vi "getDeviceParam.vi"(9 "deviceNo":i32, 10 "param":string, 11 "driver":string) -> (3 "Result":string)   [LabVIEW 2015]
uses:
  <instrlib>/niModInst/niModInst Get Installed Device Attribute (String).vi
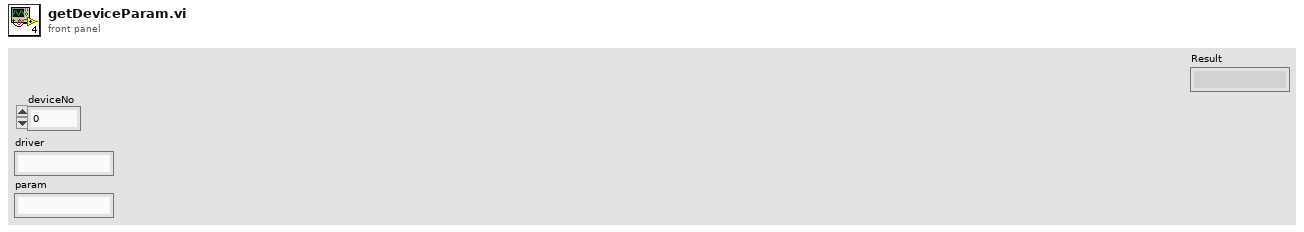
[diagram p1: front panel]
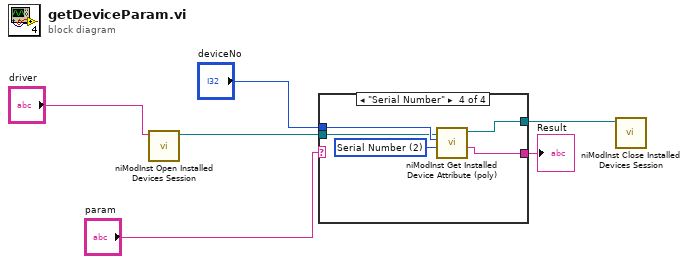
[diagram p0: block diagram]
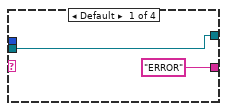
[diagram p2: hidden frame]
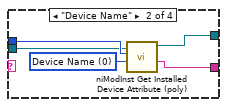
[diagram p3: hidden frame]
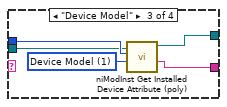
[diagram p4: hidden frame]
diagram:
  n1 = call <instrlib>:"niModInst Open Installed Devices Session.vi"("driver"="driver") -> ("session"=w5:refnum<k20>)  [unwired: 8 in, 2 out]
  n2 = case shown="\"Serial Number\"" "param" {
    tunnel: "deviceNo" -> [_ w12 w17 w22]
    tunnel: w5 -> [w7 w11 w16 w21]
    tunnel: ["ERROR" w10 w15 w20] -> w4
    tunnel: [w7 w9 w14 w19] -> w3
    frame Default {
    }
    frame "Device Name" {
      w13 = 0 items=["Device Name", "Device Model", "Serial Number"] ("attribute ID")
      n3 = call-poly <instrlib>:"niModInst Get Installed Device Attribute (poly).vi"("attribute ID"=w13, "index in"=w12, "session in"=w11) -> ("attribute value"=w10:string, "session out"=w9:refnum<k20>)  [unwired: 5 in, 2 out]
    }
    frame "Device Model" {
      w18 = 1 items=["Device Name", "Device Model", "Serial Number"] ("attribute ID")
      n4 = call-poly <instrlib>:"niModInst Get Installed Device Attribute (poly).vi"("attribute ID"=w18, "index in"=w17, "session in"=w16) -> ("attribute value"=w15:string, "session out"=w14:refnum<k20>)  [unwired: 5 in, 2 out]
    }
    frame "Serial Number" {
      w23 = 2 items=["Device Name", "Device Model", "Serial Number"] ("attribute ID")
      n5 = call-poly <instrlib>:"niModInst Get Installed Device Attribute (poly).vi"("attribute ID"=w23, "index in"=w22, "session in"=w21) -> ("attribute value"=w20:string, "session out"=w19:refnum<k20>)  [unwired: 5 in, 2 out]
    }
  }
  "Result" <- w4
  n6 = call <instrlib>:"niModInst Close Installed Devices Session.vi"("session"=w3) -> ()  [unwired: 10 in, 1 out]
